vi "Simple Edge Detection.vi"(9 "Mode":T1(ring), 11 "clk_in":bool) -> (3 "edge?":bool)   [LabVIEW 2015]
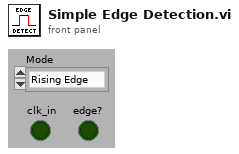
[diagram p1: front panel]
types:
  T1 = enum16{"Rising Edge", "Falling Edge", "Any Edge"}
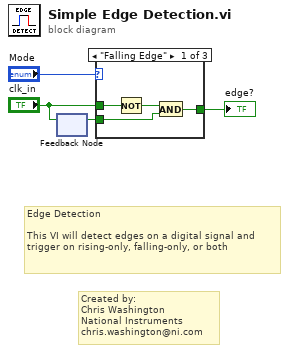
[diagram p0: block diagram]
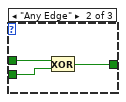
[diagram p2: hidden frame]
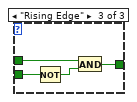
[diagram p3: hidden frame]
diagram:
  # "Created by:\nChris Washington\nNational Instruments\nchris.washington@ni.com"
  # "Edge Detection\n\nThis VI will detect edges on a digital signal and trigger on rising-only, falling-only, or both"
  n1 = feedback-in #1("clk_in") -> ()
  n2 = feedback #1() -> (w2:bool)  [unwired: 1 in]
  n3 = case shown="\"Falling Edge\"" "Mode" {
    tunnel: "clk_in" -> [w8 w11 w15]
    tunnel: [w7 w10 w14] -> w3
    tunnel: w2 -> [w5 w9 w12]
    frame "Falling Edge" {
      n4 = Not(x=w8) -> (.not. x?=w6:bool)
      n5 = And(x=w6, y=w5) -> (x .and. y?=w7:bool)
    }
    frame "Any Edge" {
      n6 = Exclusive Or(1:w9, 2:w11) -> (0:w10:bool)
    }
    frame "Rising Edge" {
      n7 = Not(x=w12) -> (.not. x?=w13:bool)
      n8 = And(x=w15, y=w13) -> (x .and. y?=w14:bool)
    }
  }
  "edge?" <- w3
